vi "MTMount_putSample_SafetySystem.vi"(8 "error in (no error)":errorcluster, 11 "Safety_System_Ctl":T1) -> (0 "error out":errorcluster, 2 "function return":i32, 3 "Safety_System_Ctl out":T1)   [LabVIEW 2018, in "SALLV_MTMount.lvlib"]
doc: "int MTMount_shm_putSample_Safety_SystemLV(MTMount_Safety_SystemLV *Safety_System_Ctl );"
uses:
  SALLV_MTMount.lvlib
  DataTypes/Safety_System.ctl
  SALLV_MTMount.so
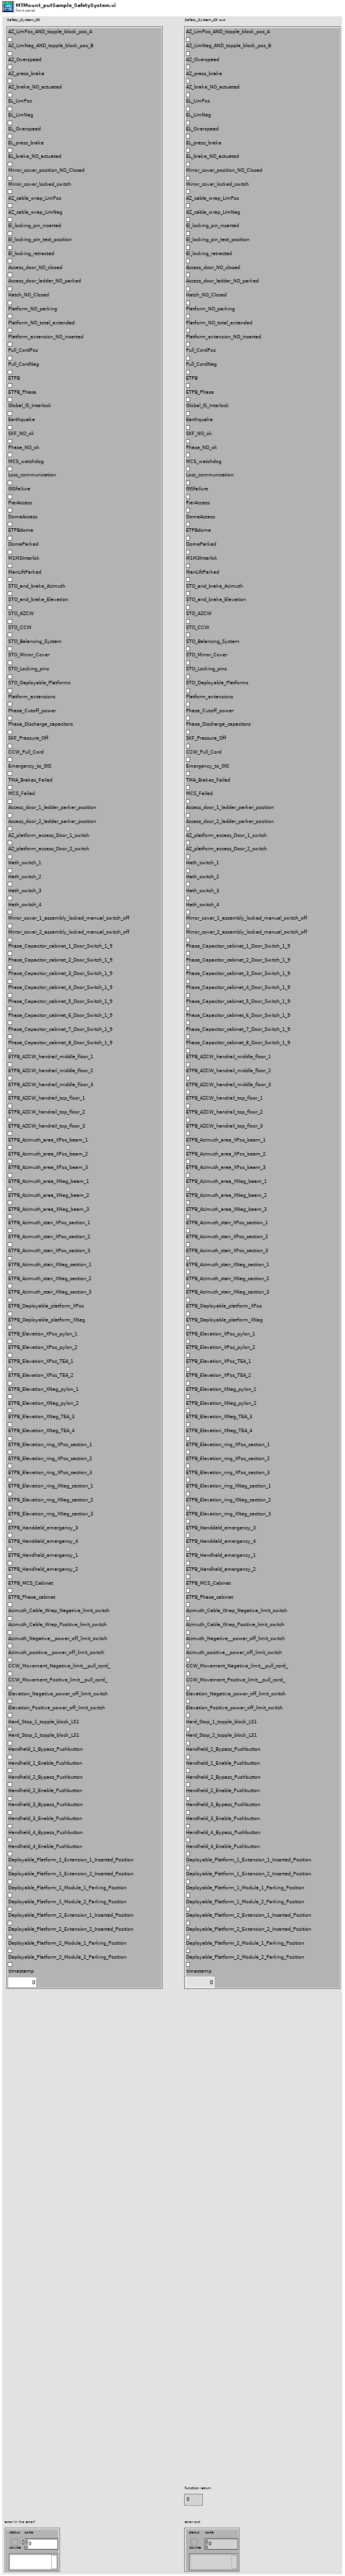
[diagram p1: front panel]
types:
  T1 = typedef "SALLV_MTMount.lvlib/Safety_System.ctl" = cluster{"AZ_LimPos_AND_topple_block_pos_A":bool, "AZ_LimNeg_AND_topple_block_pos_B":bool, "AZ_Overspeed":bool, "AZ_press_brake":bool, "AZ_brake_NO_actuated":bool, "EL_LimPos":bool, "EL_LimNeg":bool, "EL_Overspeed":bool, "EL_press_brake":bool, "EL_brake_NO_actuated":bool, "Mirror_cover_position_NO_Closed":bool, "Mirror_cover_locked_switch":bool, "AZ_cable_wrap_LimPos":bool, "AZ_cable_wrap_LimNeg":bool, "El_locking_pin_inserted":bool, "El_locking_pin_test_position":bool, "El_locking_retracted":bool, "Access_door_NO_closed":bool, "Access_door_ladder_NO_parked":bool, "Hatch_NO_Closed":bool, "Platform_NO_parking":bool, "Platform_NO_total_extended":bool, "Platform_extension_NO_inserted":bool, "Pull_CordPos":bool, "Pull_CordNeg":bool, "ETPB":bool, "ETPB_Phase":bool, "Global_IS_Interlock":bool, "Earthquake":bool, "SKF_NO_ok":bool, "Phase_NO_ok":bool, "MCS_watchdog":bool, "Loss_communication":bool, "GISfailure":bool, "PierAccess":bool, "DomeAccess":bool, "ETPBdome":bool, "DomeParked":bool, "M1M3Interlok":bool, "ManLiftParked":bool, "STO_and_brake_Azimuth":bool, "STO_and_brake_Elevation":bool, "STO_AZCW":bool, "STO_CCW":bool, "STO_Balancing_System":bool, "STO_Mirror_Cover":bool, "STO_Locking_pins":bool, "STO_Deployable_Platforms":bool, "Platform_extensions":bool, "Phase_Cutoff_power":bool, "Phase_Discharge_capacitors":bool, "SKF_Pressure_Off":bool, "CCW_Pull_Cord":bool, "Emergency_to_GIS":bool, "TMA_Brakes_Failed":bool, "MCS_Failed":bool, "Access_door_1_ladder_parker_position":bool, "Access_door_2_ladder_parker_position":bool, "AZ_platform_access_Door_1_switch":bool, "AZ_platform_access_Door_2_switch":bool, "Hath_switch_1":bool, "Hath_switch_2":bool, "Hath_switch_3":bool, "Hath_switch_4":bool, "Mirror_cover_1_assembly_locked_manual_switch_off":bool, "Mirror_cover_2_assembly_locked_manual_switch_off":bool, "Phase_Capacitor_cabinet_1_Door_Switch_1_9":bool, "Phase_Capacitor_cabinet_2_Door_Switch_1_9":bool, "Phase_Capacitor_cabinet_3_Door_Switch_1_9":bool, "Phase_Capacitor_cabinet_4_Door_Switch_1_9":bool, "Phase_Capacitor_cabinet_5_Door_Switch_1_9":bool, "Phase_Capacitor_cabinet_6_Door_Switch_1_9":bool, "Phase_Capacitor_cabinet_7_Door_Switch_1_9":bool, "Phase_Capacitor_cabinet_8_Door_Switch_1_9":bool, "ETPB_AZCW_handrail_middle_floor_1":bool, "ETPB_AZCW_handrail_middle_floor_2":bool, "ETPB_AZCW_handrail_middle_floor_3":bool, "ETPB_AZCW_handrail_top_floor_1":bool, "ETPB_AZCW_handrail_top_floor_2":bool, "ETPB_AZCW_handrail_top_floor_3":bool, "ETPB_Azimuth_area_XPos_beam_1":bool, "ETPB_Azimuth_area_XPos_beam_2":bool, "ETPB_Azimuth_area_XPos_beam_3":bool, "ETPB_Azimuth_area_XNeg_beam_1":bool, "ETPB_Azimuth_area_XNeg_beam_2":bool, "ETPB_Azimuth_area_XNeg_beam_3":bool, "ETPB_Azimuth_stair_XPos_section_1":bool, "ETPB_Azimuth_stair_XPos_section_2":bool, "ETPB_Azimuth_stair_XPos_section_3":bool, "ETPB_Azimuth_stair_XNeg_section_1":bool, "ETPB_Azimuth_stair_XNeg_section_2":bool, "ETPB_Azimuth_stair_XNeg_section_3":bool, "ETPB_Deployable_platform_XPos":bool, "ETPB_Deployable_platform_XNeg":bool, "ETPB_Elevation_XPos_pylon_1":bool, "ETPB_Elevation_XPos_pylon_2":bool, "ETPB_Elevation_XPos_TEA_1":bool, "ETPB_Elevation_XPos_TEA_2":bool, "ETPB_Elevation_XNeg_pylon_1":bool, "ETPB_Elevation_XNeg_pylon_2":bool, "ETPB_Elevation_XNeg_TEA_3":bool, "ETPB_Elevation_XNeg_TEA_4":bool, "ETPB_Elevation_ring_XPos_section_1":bool, "ETPB_Elevation_ring_XPos_section_2":bool, "ETPB_Elevation_ring_XPos_section_3":bool, "ETPB_Elevation_ring_XNeg_section_1":bool, "ETPB_Elevation_ring_XNeg_section_2":bool, "ETPB_Elevation_ring_XNeg_section_3":bool, "ETPB_Handdeld_emergency_3":bool, "ETPB_Handdeld_emergency_4":bool, "ETPB_Handheld_emergency_1":bool, "ETPB_Handheld_emergency_2":bool, "ETPB_MCS_Cabinet":bool, "ETPB_Phase_cabinet":bool, "Azimuth_Cable_Wrap_Negative_limit_switch":bool, "Azimuth_Cable_Wrap_Positive_limit_switch":bool, "Azimuth_Negative__power_off_limit_switch":bool, "Azimuth_positive__power_off_limit_switch":bool, "CCW_Movement_Negative_limit__pull_cord_":bool, "CCW_Movement_Positive_limit__pull_cord_":bool, "Elevation_Negative_power_off_limit_switch":bool, "Elevation_Positive_power_off_limit_switch":bool, "Hard_Stop_1_topple_block_LS1":bool, "Hard_Stop_2_topple_block_LS1":bool, "Handheld_1_Bypass_Pushbutton":bool, "Handheld_1_Enable_Pushbutton":bool, "Handheld_2_Bypass_Pushbutton":bool, "Handheld_2_Enable_Pushbutton":bool, "Handheld_3_Bypass_Pushbutton":bool, "Handheld_3_Enable_Pushbutton":bool, "Handheld_4_Bypass_Pushbutton":bool, "Handheld_4_Enable_Pushbutton":bool, "Deployable_Platform_1_Extension_1_Inserted_Position":bool, "Deployable_Platform_1_Extension_2_Inserted_Position":bool, "Deployable_Platform_1_Module_1_Parking_Position":bool, "Deployable_Platform_1_Module_2_Parking_Position":bool, "Deployable_Platform_2_Extension_1_Inserted_Position":bool, "Deployable_Platform_2_Extension_2_Inserted_Position":bool, "Deployable_Platform_2_Module_1_Parking_Position":bool, "Deployable_Platform_2_Module_2_Parking_Position":bool, "timestamp":dbl}
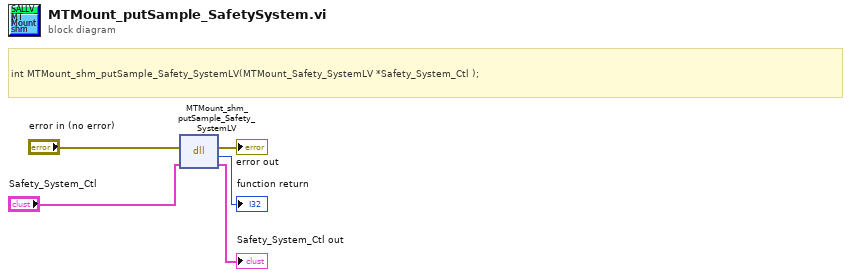
[diagram p0: block diagram]
diagram:
  # "int MTMount_shm_putSample_Safety_SystemLV(MTMount_Safety_SystemLV *Safety_System_Ctl );"
  n1 = dll-call lib="home/ttsai/Document/salApiMTMount/SALLV_MTMount/SALLV_MTMount.*" fn="MTMount_shm_putSample_Safety_SystemLV"(error in="error in (no error)", "Safety_System_Ctl"="Safety_System_Ctl") -> (error out=→"error out":errorcluster, →"function return":i32, "Safety_System_Ctl"=→"Safety_System_Ctl out":T1)  [unwired: 2 in, 1 out]
